vi "LakeShore331Read2Channel.vi"(8 "error in (no error)":errorcluster, 11 "LKS331\nGPIB Address":i16) -> (0 "error out":errorcluster, 2 "TempCryostat":dbl, 3 "TempProbe":dbl)   [LabVIEW 2014]
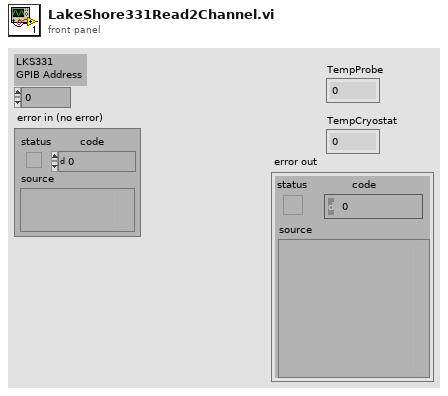
[diagram p1: front panel]
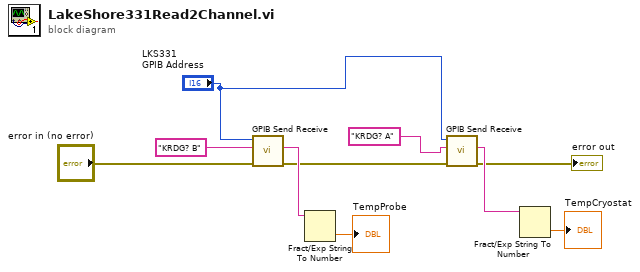
[diagram p0: block diagram]
diagram:
  n1 = call "GPIB Send Receive.vi"("error in (no error)"="error in (no error)", "data string in"="KRDG? B", "GPIB Adress"="LKS331\nGPIB Address") -> ("error out"=w3:errorcluster, "data string out"=w8:string)  [unwired: 6 in, 1 out]
  n2 = Fract/Exp String To Number(string=w8) -> (number=→"TempProbe":dbl)  [unwired: 3 in, 1 out]
  n3 = call "GPIB Send Receive.vi"("error in (no error)"=w3, "data string in"="KRDG? A", "GPIB Adress"="LKS331\nGPIB Address") -> ("error out"=→"error out":errorcluster, "data string out"=w7:string)  [unwired: 6 in, 1 out]
  n4 = Fract/Exp String To Number(string=w7) -> (number=→"TempCryostat":dbl)  [unwired: 3 in, 1 out]
